vi "create-header.vi"(11 "htmlin":string="<!DOCTYPE HTML PUBLIC \"-//W3C//DTD HTML 4.0 Transitional//EN\">\n<HTML>\n<!-- Constructed with LabVIEW Report Generation -->\n<HEAD>\n<TITLE></TITLE>\n</HEAD>\n\n<BODY>\n<div class=\"content\">\n\t<div id=\"top\">\n\t\t\t\t</div>\n\t\t\t\t<h1>MTA</h1>\n\t\t\t\t<h2>Measurements Tests and Analysis</h2>\n\t</div>Test of VI documentation in the VI documentation <BR>\n<BR>\nThese were the words of the famous physicist Albert Einstein, who went on to say that \"Knowledge is limited. Imagination encircles the world.\"<BR>\nIf you venture into the subatomic world in an attempt to unveil its inner workings, possession of all the knowledge in the world is not enough. Instead, invite your imagination to serve as a guide, because many rules as we know them no longer apply. Just like the story of Alice In Wonderland, this new world may look familiar but it is not fully comprehensible. Scales shift and matter transforms. Transitory twins appear and extra dimensions hide.<BR>\nNature has the ability to throw us the biggest surprises, so expect dramatic twists and unexpected turns; many before you have dreamed up mindÐblowing theories and crazy concepts. Some of these have prevailed against the tests of time and armies of knowledgeable critics Ð thus far.<BR>\nSomeone, sometime, somewhere, may succeed in completing these unfinished mysteries, or even rewrite the chapters entirely. The book is by no means finished.<BR><BR><BR><IMG SRC=\"LVtemp0333849524065.jpg\"  ALT=\"main.vi\"><BR><BR><BR><IMG SRC=\"LVtemp0333849524074d.jpg\" ><BR><BR><BR><BR><BR><div class=\"content\">\n\t<div id=\"top\">\n\t\t\t\t</div>\n\t\t\t\t<h1>MTA</h1>\n\t\t\t\t<h2>Measurements Tests and Analysis</h2>\n\t</div></BODY>\n</HTML>") -> (3 "replaced header":string)   [LabVIEW 2014]
panel:
  in  "relative path to css from html":string="<!DOCTYPE HTML PUBLIC \"-//W3C//DTD HTML 4.0 Transitional//EN\">\n<HTML>\n<!-- Constructed with LabVIEW Report Generation -->\n<HEAD>\n<TITLE></TITLE>\n</HEAD>\n\n<BODY>\n<div class=\"content\">\n\t<div id=\"top\">\n\t\t\t\t</div>\n\t\t\t\t<h1>MTA</h1>\n\t\t\t\t<h2>Measurements Tests and Analysis</h2>\n\t</div>Test of VI documentation in the VI documentation <BR>\n<BR>\nThese were the words of the famous physicist Albert Einstein, who went on to say that \"Knowledge is limited. Imagination encircles the world.\"<BR>\nIf you venture into the subatomic world in an attempt to unveil its inner workings, possession of all the knowledge in the world is not enough. Instead, invite your imagination to serve as a guide, because many rules as we know them no longer apply. Just like the story of Alice In Wonderland, this new world may look familiar but it is not fully comprehensible. Scales shift and matter transforms. Transitory twins appear and extra dimensions hide.<BR>\nNature has the ability to throw us the biggest surprises, so expect dramatic twists and unexpected turns; many before you have dreamed up mindÐblowing theories and crazy concepts. Some of these have prevailed against the tests of time and armies of knowledgeable critics Ð thus far.<BR>\nSomeone, sometime, somewhere, may succeed in completing these unfinished mysteries, or even rewrite the chapters entirely. The book is by no means finished.<BR><BR><BR><IMG SRC=\"LVtemp0333849524065.jpg\"  ALT=\"main.vi\"><BR><BR><BR><IMG SRC=\"LVtemp0333849524074d.jpg\" ><BR><BR><BR><BR><BR><div class=\"content\">\n\t<div id=\"top\">\n\t\t\t\t</div>\n\t\t\t\t<h1>MTA</h1>\n\t\t\t\t<h2>Measurements Tests and Analysis</h2>\n\t</div></BODY>\n</HTML>"
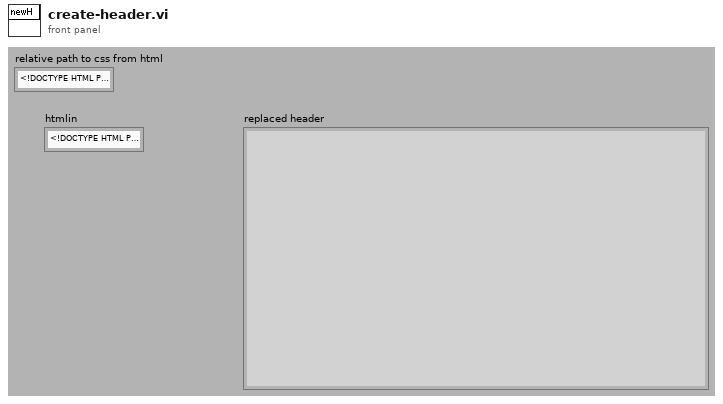
[diagram p1: front panel]
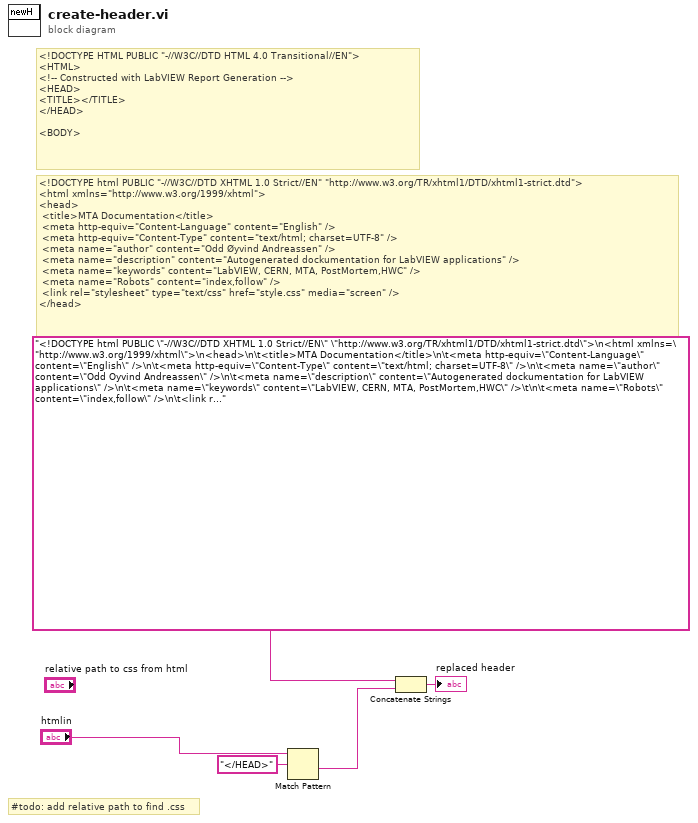
[diagram p0: block diagram]
diagram:
  # "#todo: add relative path to find .css"
  # "<!DOCTYPE html PUBLIC \"-//W3C//DTD XHTML 1.0 Strict//EN\" \"http://www.w3.org/TR/xhtml1/DTD/xhtml1-strict.dtd\">\n<html xmlns=\"http://www.w3.org/1999/xhtml\">\n<head>\n\t<title>MTA Documentation</title>\n\t<meta http-equiv=\"Content-Language\" content=\"English\" />\n\t<meta http-equiv=\"Content-Type\" content=\"text/html; charset=UTF-8\" />\n\t<meta name=\"author\" content=\"Odd Øyvind Andreassen\" />\n\t<meta name=\"description\" content=\"Autogenerated dockumentation for LabVIEW applications\" />\n\t<meta name=\"keywords\" content=\"LabVIEW, CERN, MTA, PostMortem,HWC\" />\t\n\t<meta name=\"Robots\" content=\"index,follow\" />\n\t<link rel=\"stylesheet\" type=\"text/css\" href=\"style.css\" media=\"screen\" />\n</head>"
  # "<!DOCTYPE HTML PUBLIC \"-//W3C//DTD HTML 4.0 Transitional//EN\">\n<HTML>\n<!-- Constructed with LabVIEW Report Generation -->\n<HEAD>\n<TITLE></TITLE>\n</HEAD>\n\n<BODY>"
  n1 = Match Pattern(string="htmlin", regular expression="</HEAD>") -> (after substring=w4:string)  [unwired: 4 out]
  n2 = Concatenate Strings("<!DOCTYPE html PUBLIC \"-//W3C//DTD XHTML 1.0 Strict//EN\" \"http://www.w3.org/TR/xhtml1/DTD/xhtml1-strict.dtd\">\n<html xmlns=\"http://www.w3.org/1999/xhtml\">\n<head>\n\t<title>MTA Documentation</title>\n\t<meta http-equiv=\"Content-Language\" content=\"English\" />\n\t<meta http-equiv=\"Content-Type\" content=\"text/html; charset=UTF-8\" />\n\t<meta name=\"author\" content=\"Odd Oyvind Andreassen\" />\n\t<meta name=\"description\" content=\"Autogenerated dockumentation for LabVIEW applications\" />\n\t<meta name=\"keywords\" content=\"LabVIEW, CERN, MTA, PostMortem,HWC\" />\t\n\t<meta name=\"Robots\" content=\"index,follow\" />\n\t<link rel=\"stylesheet\" type=\"text/css\" href=\"../../CSS/style.css\" media=\"screen\" />\n</head>\n\n<div class=\"content\">\n\t<div id=\"top\">\n\t\t\t\t<h4>MTA</h4>\n\t\t\t\t<h5>Measurements Tests and Analysis</h5>\n     <br>\n     <br>\n    <FORM><INPUT TYPE=\"button\" VALUE=\"<-- back\" onClick=\"history.go(-1);return true;\"></FORM>\n </div>\n</div>", w4) -> (→"replaced header":string)
